vi "LoadPatientInfo_Profile.vi"(8 "error in":errorcluster, 11 "DataPatientPath":path) -> (0 "error out":errorcluster, 3 "profile":T1)   [LabVIEW 2013, in "main.lvlib"]
uses:
  main.lvlib
  Controls/date_specific_info.ctl
  Globals/DataPathGlobalVariable.vi
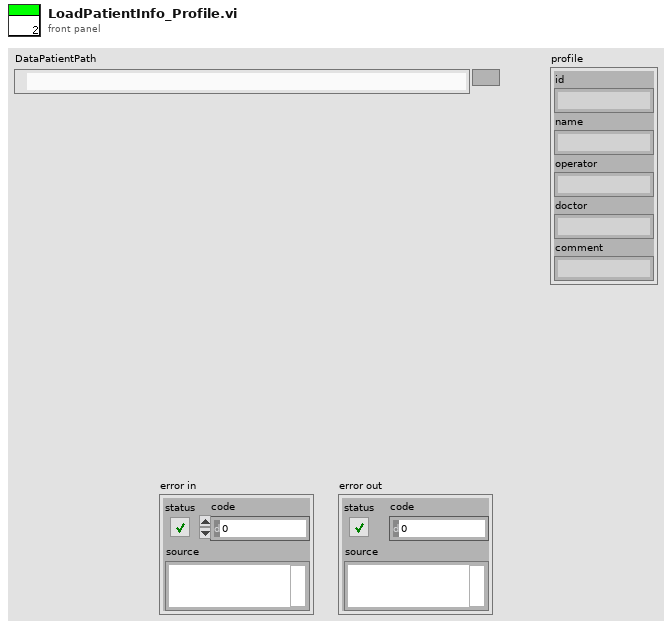
[diagram p1: front panel]
types:
  T1 = cluster{"id":string, "name":string, "operator":string, "doctor":string, "comment":string}
  T2 = enum16{"open", "replace", "create", "open or create", "replace or create", "replace or create with confirmation"}
  T3 = typedef "main.lvlib/date_specific_info.ctl" = cluster{"profile":cluster{"id":string, "name":string, "operator":string, "doctor":string, "comment":string}, "hospital":cluster{"name":string, "department":string, "address":string}, "palpation":cluster{"right":string, "left":string}, "Armpressure Right":cluster{"sys":dbl, "dia":dbl, "puls":dbl, "date":string, "time":string, "code":string, "serial":string, "temp":dbl, "activity":string}[], "Armpressure Left":cluster{"sys":dbl, "dia":dbl, "puls":dbl, "date":string, "time":string, "code":string, "serial":string, "temp":dbl, "activity":string}[]}
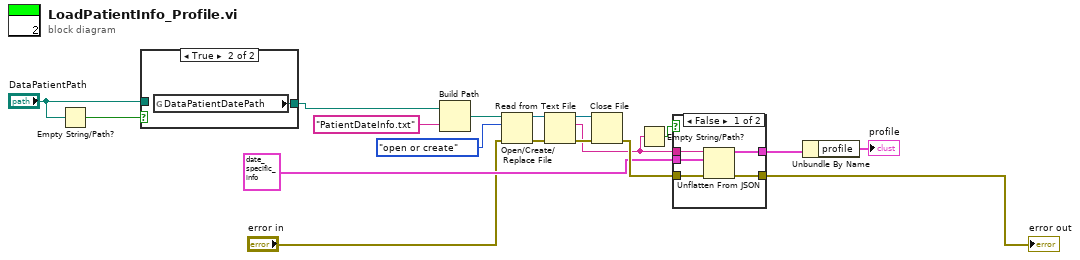
[diagram p0: block diagram]
diagram:
  n1 = Empty String/Path?(string/path="DataPatientPath") -> (empty?=w18:bool)
  n2 = case shown="True" w18 {
    tunnel: [w19 w20] -> w1
    tunnel: "DataPatientPath" -> [w19 _]
    frame False {
    }
    frame True {
      n3 = global read "DataPathGlobalVariable.vi" "DataPatientDatePath"() -> (w20:path)
    }
  }
  n4 = Build Path(base path=w1, name or relative path="PatientDateInfo.txt") -> (appended path=w13:path)
  n5 = Open/Create/Replace File(file path (use dialog)=w13, error in="error in", operation (0:open)=T2."open or create") -> (refnum out=w15:refnum<file>, error out=w14:errorcluster)  [unwired: 3 in, 1 out]
  n6 = Read from Text File(file (use dialog)=w15, error in=w14) -> (refnum out=w11:refnum<file>, text=w7:string, error out=w10:errorcluster)  [unwired: 2 in, 1 out]
  n7 = Close File(refnum=w11, error in=w10) -> (error out=w8:errorcluster)  [unwired: 1 out]
  n8 = Empty String/Path?(string/path=w7) -> (empty?=w9:bool)
  n9 = case shown="False" w9 {
    tunnel: w7 -> [w25 _]
    tunnel: w8 -> [w24 w27]
    tunnel: [w23 w26] -> w6
    tunnel: [w22 w27] -> w4
    tunnel: T3 {"profile"={"id"="", "name"="", "operator"="", "doctor"="", "comment"=""}, "hospital"={"name"="", "department"="", "address"=""}, "palpation"={"right"="", "left"=""}, "Armpressure Right"=[], "Armpressure Left"=[]} ("date_specific_info") -> [w21 w26]
    frame False {
      n10 = Unflatten From JSON(JSON string=w25, type and defaults=w21, error in (no error)=w24) -> (value=w23:T3, error out=w22:errorcluster)  [unwired: 4 in]
    }
    frame True {
    }
  }
  "error out" <- w4
  n11 = Unbundle By Name(w6) -> ("profile"=→"profile":T1)
